vi "Facade.vi"(0 "Data In":T29={"Waveform"={"Type"=enum."Tone", "Tone"={"Frequency (kHz)"=0.0, "Last Freq"=0.0, "Last Phase"=0.0}, "Pulse Train"={"Pulse width (us)"=0.0, "Pulse rate (Hz)"=0.0, "Gap (ms)"=0.0, "Polarity"=enum."POS", "PT State"={"Template"=[], "Nperiod"=0, "Index"=0, "Pulse Rate (Hz)"=0.0, "Phase (cycles)"=0.0, "Noff"=0}, "Asynch"=FALSE}, "Noise"={"InvFilt"=FALSE, "Noise"=[], "CurPt"=0, "Aweight"=FALSE, "Seed"=0, "afile"=path ""}, "File"={"Filename"=path "", "Signal"=[], "Channel"=0, "stream"=FALSE, "offset"=0, "nreps"=0, "loops"=0, "Randomize"=FALSE, "order"=[], "Seed"=0, "Tokens"=0}, "FMSweep"={"Rate (oct/s)"=0.0, "Fmin (Hz)"=0.0, "Fmax (Hz)"=0.0, "Ramp (ms)"=0.0, "Linear"=FALSE}, "Chirp Train"={"Params"={"Fmin (kHz)"=4.0, "Fmax (kHz)"=64.0, "Compensate"=FALSE, "Duration (ms)"=2.0}, "Data"={"WF"=[]}}, "Complex Tone"={"Params"={"F0 (Hz)"=0.0, "Band"={"Flow (Hz)"=0.0, "Fhigh (Hz)"=0.0}, "Phase"=enum."Cosine", "Min F0 (Hz)"=0.0, "Max F0 (Hz)"=0.0, "ContinRandPhase"=FALSE, "Max peak factor"=inf, "Max mod depth"=2.0, "MinHarmNum"=0, "MaxHarmNum"=0, "Level Mode"=enum."per component", "% jitter"=0.0}, "Data"={"Ncomp"=0, "MinHarm"=0, "Phase"=[], "Amplitude"=[], "Npts/frame"=0, "Last F0"=0.0, "Fmin"=0.0, "Fmax"=0.0, "Lslope"=0.0, "randphase"=FALSE, "overall rms"=FALSE, "fmult"=[], "jittered"=FALSE}}, "Moving Ripple"={"Params"={"Fmin"=0.0, "Fmax"=0.0, "Density"=0.0, "Velocity"=0.0, "Depth"=0.0, "Phase"=0.0, "Comp/oct"=0}, "Data"={"Freq"=[], "A"=[], "phase"=[], "Phase"=0.0}}}, "Filter"={"Type"=enum."Lowpass", "CF (kHz)"=0.0, "BW (kHz)"=0.0, "Cascade"=FALSE, "Quadrature"=FALSE, "Scale Factor"=0.0, "Stages"=[], "Class"=enum."Elliptic", "Order"=0, "BWUnits"=enum."Linear"}, "Burst"={"Active"=FALSE, "Delay (ms)"=0.0, "Duration (ms)"=50.0, "Ramp (ms)"=5.0, "Rate (Hz)"=0.0, "Trepeat (ms)"=0.0, "Repeat"=FALSE}, "Level"={"Level"=0.0, "Units"=enum."dB atten", "Max"=0.0, "Multiplier"=0.0, "Cal File"=path "", "Cal"={"Freq (Hz)"=[], "Mag (dB SPL)"=[], "Phase (deg)"=[]}}, "Name"="", "Advanced"={"Rep Mask"="", "AltPol"=FALSE, "Var"="", "Expr"="", "Persist"=FALSE}, "SAM"={"Active"=FALSE, "Frequency (Hz)"=0.0, "Depth"=0.0, "Init Phase (cycles)"=0.0, "phase (degrees)"=0.0, "Asynch"=FALSE}} {"Filter"."Stages"."IIR Filter"."Forward Coefficients" format="%.4f"; "Filter"."Stages"."IIR Filter"."Reverse Coefficients" format="%.4f"}, 2 "Display State In":T27={"Update"=FALSE, "Show advanced"=FALSE, "Fs (Hz)"=100000.0, "Show persist"=FALSE}, 3 "Container State":T28) -> (6 "Data Out":T29={"Waveform"={"Type"=enum."Tone", "Tone"={"Frequency (kHz)"=0.0, "Last Freq"=0.0, "Last Phase"=0.0}, "Pulse Train"={"Pulse width (us)"=0.0, "Pulse rate (Hz)"=0.0, "Gap (ms)"=0.0, "Polarity"=enum."POS", "PT State"={"Template"=[], "Nperiod"=0, "Index"=0, "Pulse Rate (Hz)"=0.0, "Phase (cycles)"=0.0, "Noff"=0}, "Asynch"=FALSE}, "Noise"={"InvFilt"=FALSE, "Noise"=[], "CurPt"=0, "Aweight"=FALSE, "Seed"=0, "afile"=path ""}, "File"={"Filename"=path "", "Signal"=[], "Channel"=0, "stream"=FALSE, "offset"=0, "nreps"=0, "loops"=0, "Randomize"=FALSE, "order"=[], "Seed"=0, "Tokens"=0}, "FMSweep"={"Rate (oct/s)"=0.0, "Fmin (Hz)"=0.0, "Fmax (Hz)"=0.0, "Ramp (ms)"=0.0, "Linear"=FALSE}, "Chirp Train"={"Params"={"Fmin (kHz)"=4.0, "Fmax (kHz)"=64.0, "Compensate"=FALSE, "Duration (ms)"=2.0}, "Data"={"WF"=[]}}, "Complex Tone"={"Params"={"F0 (Hz)"=0.0, "Band"={"Flow (Hz)"=0.0, "Fhigh (Hz)"=0.0}, "Phase"=enum."Cosine", "Min F0 (Hz)"=0.0, "Max F0 (Hz)"=0.0, "ContinRandPhase"=FALSE, "Max peak factor"=inf, "Max mod depth"=2.0, "MinHarmNum"=0, "MaxHarmNum"=0, "Level Mode"=enum."per component", "% jitter"=0.0}, "Data"={"Ncomp"=0, "MinHarm"=0, "Phase"=[], "Amplitude"=[], "Npts/frame"=0, "Last F0"=0.0, "Fmin"=0.0, "Fmax"=0.0, "Lslope"=0.0, "randphase"=FALSE, "overall rms"=FALSE, "fmult"=[], "jittered"=FALSE}}, "Moving Ripple"={"Params"={"Fmin"=0.0, "Fmax"=0.0, "Density"=0.0, "Velocity"=0.0, "Depth"=0.0, "Phase"=0.0, "Comp/oct"=0}, "Data"={"Freq"=[], "A"=[], "phase"=[], "Phase"=0.0}}}, "Filter"={"Type"=enum."Lowpass", "CF (kHz)"=0.0, "BW (kHz)"=0.0, "Cascade"=FALSE, "Quadrature"=FALSE, "Scale Factor"=0.0, "Stages"=[], "Class"=enum."Elliptic", "Order"=0, "BWUnits"=enum."Linear"}, "Burst"={"Active"=FALSE, "Delay (ms)"=0.0, "Duration (ms)"=50.0, "Ramp (ms)"=5.0, "Rate (Hz)"=0.0, "Trepeat (ms)"=0.0, "Repeat"=FALSE}, "Level"={"Level"=0.0, "Units"=enum."dB atten", "Max"=0.0, "Multiplier"=0.0, "Cal File"=path "", "Cal"={"Freq (Hz)"=[], "Mag (dB SPL)"=[], "Phase (deg)"=[]}}, "Name"="", "Advanced"={"Rep Mask"="", "AltPol"=FALSE, "Var"="", "Expr"="", "Persist"=FALSE}, "SAM"={"Active"=FALSE, "Frequency (Hz)"=0.0, "Depth"=0.0, "Init Phase (cycles)"=0.0, "phase (degrees)"=0.0, "Asynch"=FALSE}} {"Filter"."Stages"."IIR Filter"."Forward Coefficients" format="%.4f"; "Filter"."Stages"."IIR Filter"."Reverse Coefficients" format="%.4f"}, 7 "Display State Out":T27={"Update"=FALSE, "Show advanced"=FALSE, "Fs (Hz)"=100000.0, "Show persist"=FALSE}, 8 "Action":T26)   [LabVIEW 2020, in "Stimulus Channel (Full).xctl"]
uses:
  Stimulus Channel (Full).xctl
  Full Stimulus Channel Data.ctl
  Waveform XCtl/Waveform Data.ctl
  Waveform XCtl/Waveform Enum.ctl
  Waveform VIs/Tone VIs/Tone Params.ctl
  Waveform VIs/Pulse Train VIs/Pulse Train Params.ctl
  Waveform VIs/Pulse Train VIs/Pulse Polarity.ctl
  Waveform VIs/Pulse Train VIs/PT-Continuous State.ctl
  Waveform VIs/Noise VIs/Noise Params.ctl
  Waveform VIs/File VIs/StimFile-Params.ctl
  Waveform VIs/FM Sweep VIs/FM Sweep Params.ctl
  Waveform VIs/Chirp Train VIs/Chirp Train.ctl
  Waveform VIs/Chirp Train VIs/Chirp Train Params.ctl
  Waveform VIs/Complex Tone VIs/CT-Params.ctl
  Waveform VIs/Complex Tone VIs/CT-Phase Enum.ctl
  Waveform VIs/Complex Tone VIs/CT-Runtime Data.ctl
  Waveform VIs/Moving Ripple VIs/Moving Ripple.ctl
  Waveform VIs/Moving Ripple VIs/Moving Ripple.Params.ctl
  Waveform VIs/Moving Ripple VIs/Moving Ripple.Data.ctl
  Advanced Filter XCtl/Filter Data.ctl
  Filter VIs/Filter-Bandwidth Units.ctl
  Burst XCtl/Burst Data.ctl
  Level XCtl/Level Data.ctl
  Level XCtl/Level Units.ctl
  Advanced Options XCtl/Advanced Stimulus Options.ctl
  Modulation VIs/SAM VIs/SAM Params.ctl
  <vilib>/_xctls/Container State.ctl
  State.ctl
  <vilib>/_xctls/Action.ctl
  Advanced Filter XCtl/Advanced Filter XCtl.xctl
  Level XCtl/Level XCtl.xctl
  Burst XCtl/Burst Control.xctl
  Waveform XCtl/Waveform XCtl.xctl
  Advanced Options XCtl/Advanced Stimulus Options.xctl
  <vilib>/_xctls/XControlSupport.lvlib
panel:
  out "SAM-dependent display":bool
  out "waveform-dependent display":bool
  out "update max level":bool
  in  "Tab Control":T1(tab)=enum."Filtering"
  in  "Waveform":T18(xcontrol)
  in  "Level":T20(xcontrol)
  in  "Gate":T21(xcontrol)
  in  "SAM":T22
  in  "Filter":T24(xcontrol)
  in  "Advanced":T25(xcontrol)
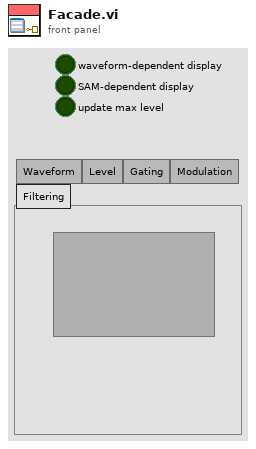
[diagram p1: front panel]
types:
  T1 = enum32{"Waveform", "Level", "Gating", "Modulation", "Filtering", "Advanced"}
  T2 = typedef "Waveform Enum.ctl" = enum16{"OFF", "Tone", "Noise", "Pulse Train", "File", "FM Sweep", "Chirp Train", "Complex Tone", "FM Tone", "Moving Ripple"}
  T3 = typedef "Tone Params.ctl" = cluster{"Frequency (kHz)":dbl, "Last Freq":dbl, "Last Phase":dbl}
  T4 = typedef "Pulse Train Params.ctl" = cluster{"Pulse width (us)":dbl, "Pulse rate (Hz)":dbl, "Gap (ms)":dbl, "Polarity":T5, "PT State":T6, "Asynch":bool}
  T5 = typedef "Pulse Polarity.ctl" = enum16{"POS", "NEG", "POS-NEG", "NEG-POS"}
  T6 = typedef "PT-Continuous State.ctl" = cluster{"Template":dbl[], "Nperiod":i32, "Index":i32, "Pulse Rate (Hz)":dbl, "Phase (cycles)":dbl, "Noff":i32}
  T7 = typedef "Noise Params.ctl" = cluster{"InvFilt":bool, "Noise":dbl[], "CurPt":i32, "Aweight":bool, "Seed":i32, "afile":path}
  T8 = typedef "StimFile-Params.ctl" = cluster{"Filename":path, "Signal":dbl[], "Channel":i32, "stream":bool, "offset":i32, "nreps":i32, "loops":i32, "Randomize":bool, "order":i32[], "Seed":i32, "Tokens":i32}
  T9 = typedef "FM Sweep Params.ctl" = cluster{"Rate (oct/s)":dbl, "Fmin (Hz)":dbl, "Fmax (Hz)":dbl, "Ramp (ms)":dbl, "Linear":bool}
  T10 = typedef "Chirp Train.ctl" = cluster{"Params":T11, "Data":cluster{"WF":dbl[]}}
  T11 = typedef "Chirp Train Params.ctl" = cluster{"Fmin (kHz)":dbl, "Fmax (kHz)":dbl, "Compensate":bool, "Duration (ms)":dbl}
  T12 = typedef "CT-Params.ctl" = cluster{"F0 (Hz)":dbl, "Band":cluster{"Flow (Hz)":dbl, "Fhigh (Hz)":dbl}, "Phase":T13, "Min F0 (Hz)":dbl, "Max F0 (Hz)":dbl, "ContinRandPhase":bool, "Max peak factor":dbl, "Max mod depth":dbl, "MinHarmNum":i32, "MaxHarmNum":i32, "Level Mode":enum16{"per component", "overall rms"}, "% jitter":dbl}
  T13 = typedef "CT-Phase Enum.ctl" = enum16{"Cosine", "Random", "Alternating"}
  T14 = typedef "CT-Runtime Data.ctl" = cluster{"Ncomp":i32, "MinHarm":i32, "Phase":dbl[], "Amplitude":dbl[], "Npts/frame":i32, "Last F0":dbl, "Fmin":dbl, "Fmax":dbl, "Lslope":dbl, "randphase":bool, "overall rms":bool, "fmult":dbl[], "jittered":bool}
  T15 = typedef "Moving Ripple.ctl" = cluster{"Params":T16, "Data":T17}
  T16 = typedef "Moving Ripple.Params.ctl" = cluster{"Fmin":dbl, "Fmax":dbl, "Density":dbl, "Velocity":dbl, "Depth":dbl, "Phase":dbl, "Comp/oct":i32}
  T17 = typedef "Moving Ripple.Data.ctl" = cluster{"Freq":dbl[], "A":dbl[], "phase":dbl[], "Phase":dbl}
  T18 = cluster{"Type":T2, "Tone":T3, "Pulse Train":T4, "Noise":T7, "File":T8, "FMSweep":T9, "Chirp Train":T10, "Complex Tone":cluster{"Params":T12, "Data":T14}, "Moving Ripple":T15}
  T19 = typedef "Level Units.ctl" = enum16{"dB atten", "dB SPL", "dB re 1 Vrms", "dB V/Hz½", "mW", "dB HL", "Volts", "dB mW"}
  T20 = cluster{"Level":dbl, "Units":T19, "Max":dbl, "Multiplier":dbl, "Cal File":path, "Cal":cluster{"Freq (Hz)":dbl[], "Mag (dB SPL)":dbl[], "Phase (deg)":dbl[]}}
  T21 = cluster{"Active":bool, "Delay (ms)":dbl, "Duration (ms)":dbl, "Ramp (ms)":dbl, "Rate (Hz)":dbl, "Trepeat (ms)":dbl, "Repeat":bool}
  T22 = cluster{"Active":bool, "Frequency (Hz)":dbl, "Depth (0-1)":dbl, "Phase (cycles)":dbl, "phase":dbl, "Asynch":bool}
  T23 = typedef "Filter-Bandwidth Units.ctl" = enum16{"Linear", "Octaves", "Min-Max"}
  T24 = cluster{"Type":enum16{"Lowpass", "Highpass", "Bandpass", "Bandstop", "OFF"}, "CF (kHz)":dbl, "BW (kHz)":dbl, "Cascade":bool, "Quadrature":bool, "Scale Factor":dbl, "Stages":cluster{"IIR Filter":cluster{"filter structure":enum32{"IIR 2nd Order", "IIR 4th Order"}, "Reverse Coefficients":dbl[], "Forward Coefficients":dbl[]}, "State":dbl[]}[], "Class":enum16{"Elliptic", "Butterworth"}, "Order":i32, "BWUnits":T23}
  T25 = cluster{"Rep Mask":string, "AltPol":bool, "Var":string, "Expr":string, "Persist":bool}
  T26 = typedef "XControlSupport.lvlib/Action.ctl" = cluster{"Data Changed?":bool, "State Changed?":bool, "Action Name":string}
  T27 = typedef "Stimulus Channel (Full).xctl/State.ctl" = cluster{"Update":bool, "Show advanced":bool, "Fs (Hz)":dbl, "Show persist":bool}
  T28 = typedef "XControlSupport.lvlib/Container State.ctl" = cluster{"Indicator?":bool, "Run Mode?":bool, " Refnum":refnum<vi>}
  T29 = typedef "Stimulus Channel (Full).xctl/Full Stimulus Channel Data.ctl" = cluster{"Waveform":T30, "Filter":T31, "Burst":T32, "Level":T33, "Name":string, "Advanced":T34, "SAM":T35}
  T30 = typedef "Waveform XCtl.xctl/Waveform Data.ctl" = cluster{"Type":T2, "Tone":T3, "Pulse Train":T4, "Noise":T7, "File":T8, "FMSweep":T9, "Chirp Train":T10, "Complex Tone":cluster{"Params":T12, "Data":T14}, "Moving Ripple":T15}
  T31 = typedef "Advanced Filter XCtl.xctl/Filter Data.ctl" = cluster{"Type":enum16{"Lowpass", "Highpass", "Bandpass", "Bandstop", "OFF"}, "CF (kHz)":dbl, "BW (kHz)":dbl, "Cascade":bool, "Quadrature":bool, "Scale Factor":dbl, "Stages":cluster{"IIR Filter":cluster{"filter structure":enum32{"IIR 2nd Order", "IIR 4th Order"}, "Reverse Coefficients":dbl[], "Forward Coefficients":dbl[]}, "State":dbl[]}[], "Class":enum16{"Elliptic", "Butterworth"}, "Order":i32, "BWUnits":T23}
  T32 = typedef "Burst Control.xctl/Burst Data.ctl" = cluster{"Active":bool, "Delay (ms)":dbl, "Duration (ms)":dbl, "Ramp (ms)":dbl, "Rate (Hz)":dbl, "Trepeat (ms)":dbl, "Repeat":bool}
  T33 = typedef "Level XCtl.xctl/Level Data.ctl" = cluster{"Level":dbl, "Units":T19, "Max":dbl, "Multiplier":dbl, "Cal File":path, "Cal":cluster{"Freq (Hz)":dbl[], "Mag (dB SPL)":dbl[], "Phase (deg)":dbl[]}}
  T34 = typedef "Advanced Stimulus Options.xctl/Advanced Stimulus Options.ctl" = cluster{"Rep Mask":string, "AltPol":bool, "Var":string, "Expr":string, "Persist":bool}
  T35 = typedef "SAM Params.ctl" = cluster{"Active":bool, "Frequency (Hz)":dbl, "Depth":dbl, "Init Phase (cycles)":dbl, "phase (degrees)":dbl, "Asynch":bool}
  T36 = enum32{"Waveform", "Level", "Gating", "Modulation", "Filtering"}
  T37 = enum16{"Lowpass", "Highpass", "Bandpass", "Bandstop", "OFF"}
  T38 = enum8{"Enabled", "Disabled", "Disabled and Grayed Out"}
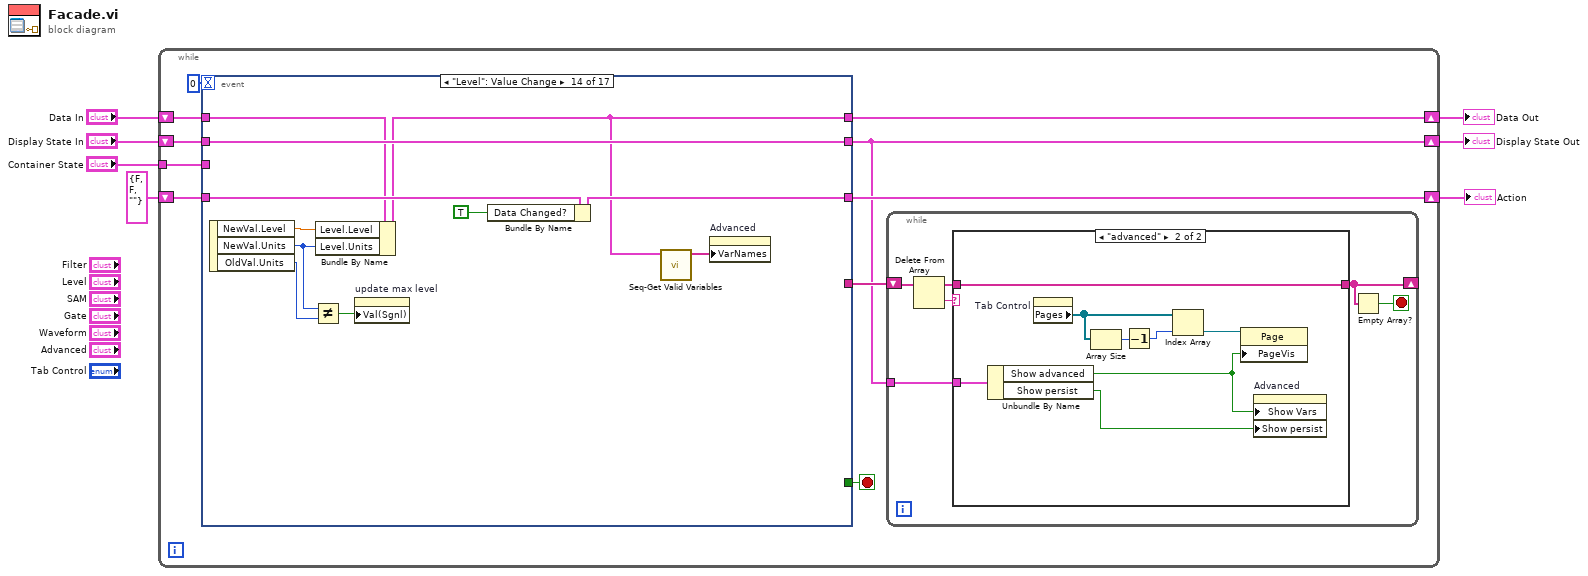
[diagram p0: block diagram]
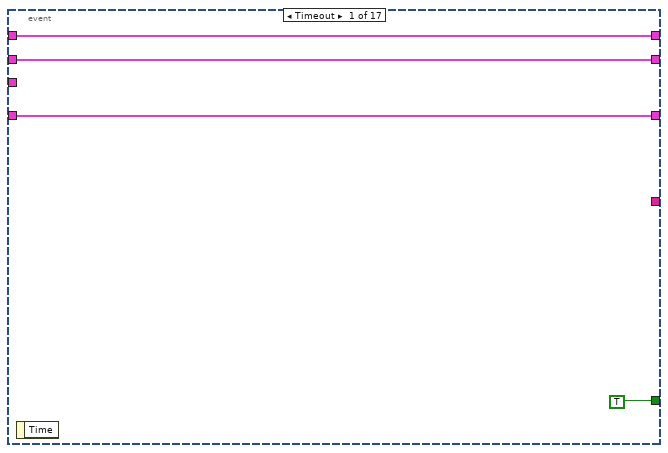
[diagram p3: hidden frame]
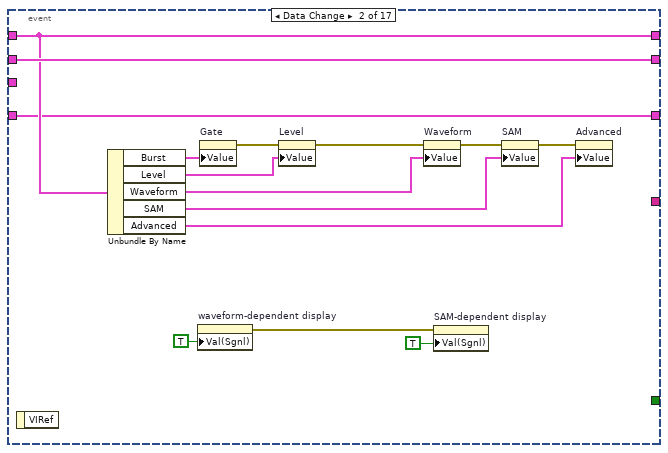
[diagram p4: hidden frame]
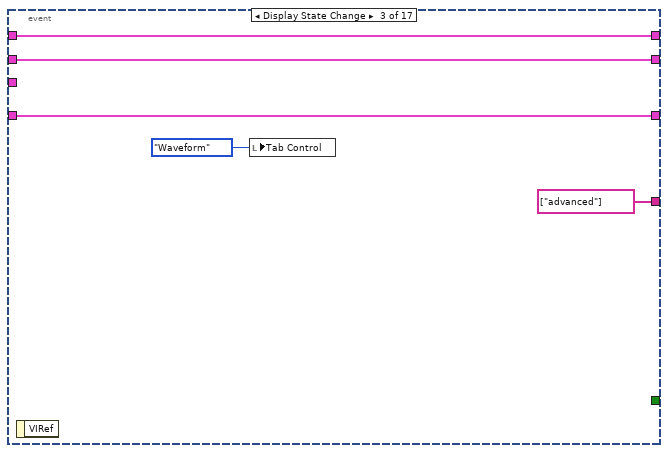
[diagram p5: hidden frame]
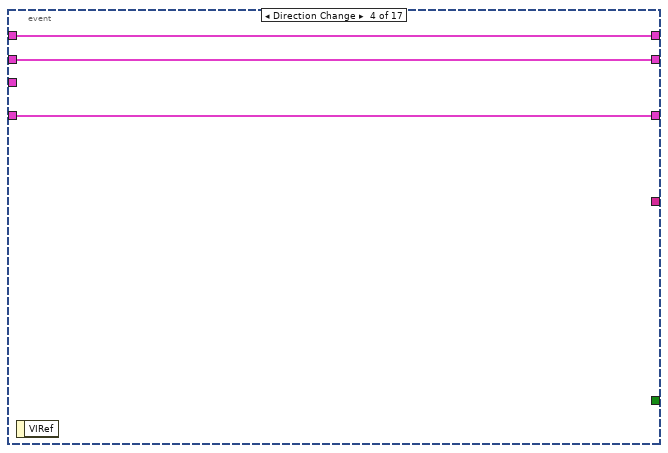
[diagram p6: hidden frame]
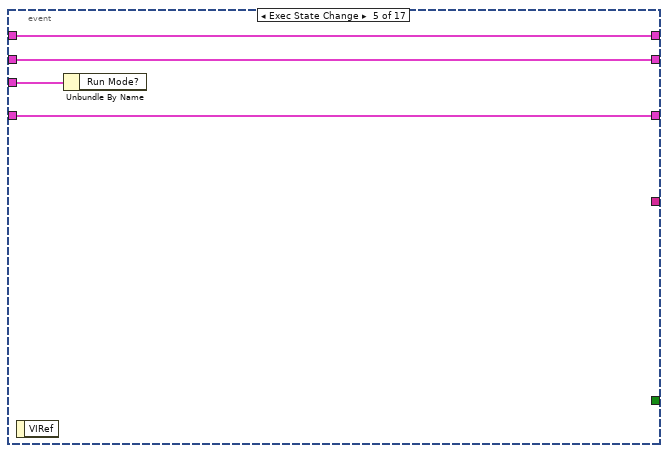
[diagram p7: hidden frame]
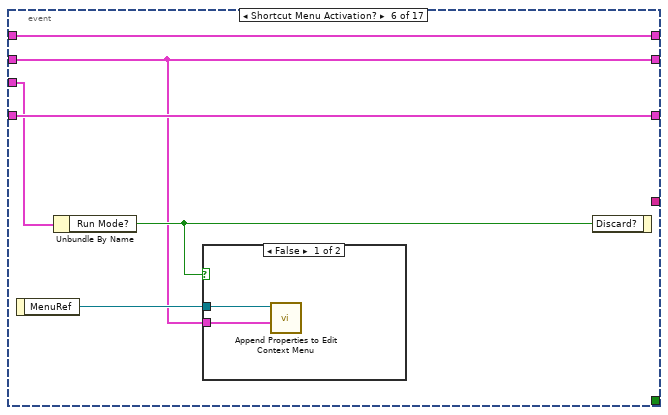
[diagram p8: hidden frame]
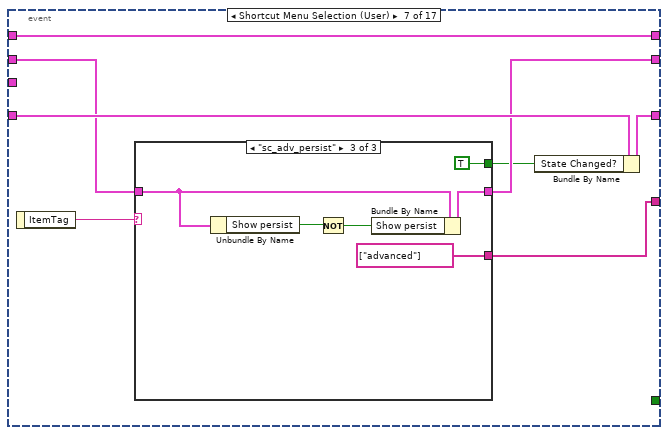
[diagram p10: hidden frame]
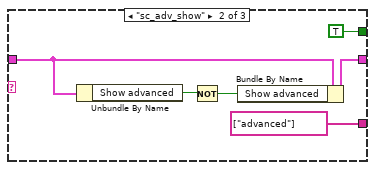
[diagram p12: hidden frame]
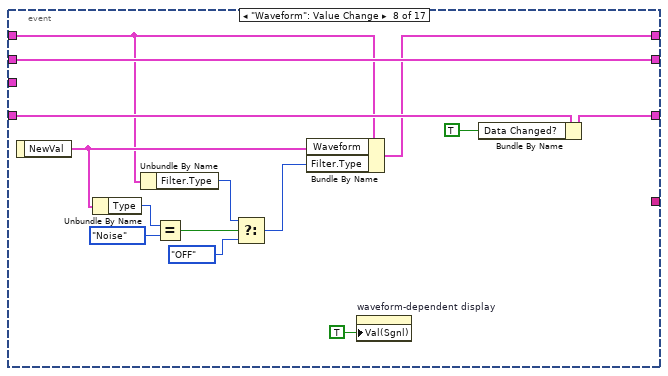
[diagram p13: hidden frame]
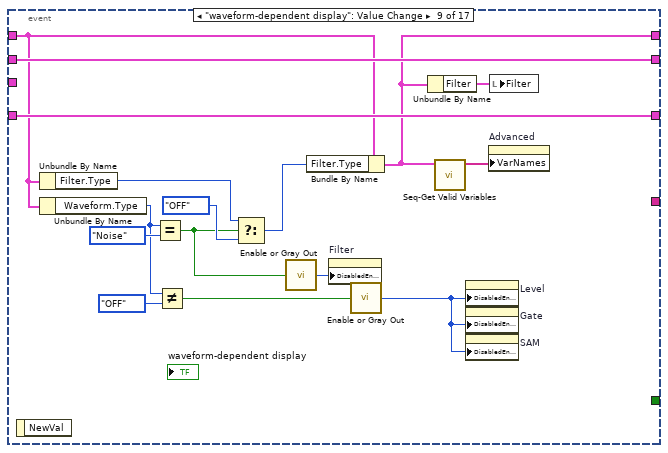
[diagram p14: hidden frame]
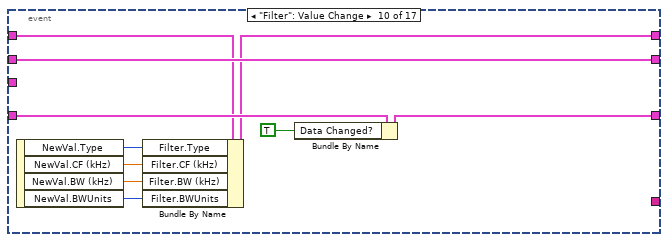
[diagram p15: hidden frame]
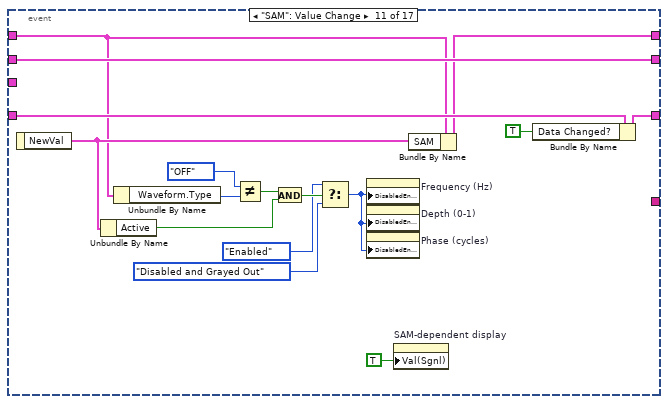
[diagram p16: hidden frame]
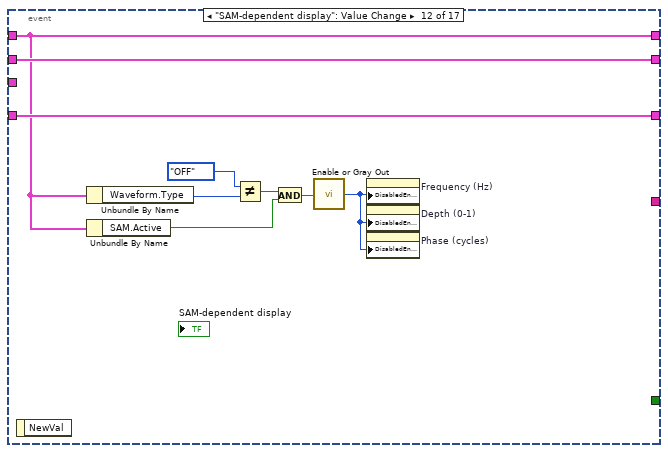
[diagram p17: hidden frame]
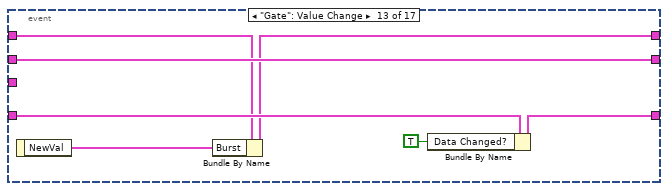
[diagram p18: hidden frame]
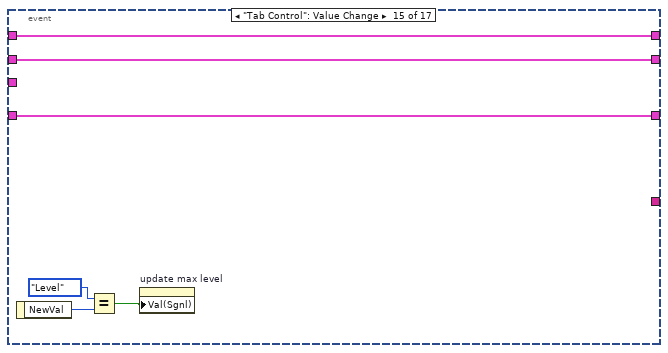
[diagram p19: hidden frame]
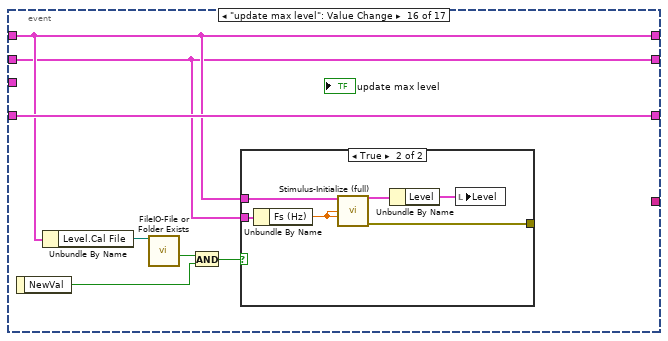
[diagram p20: hidden frame]
diagram:
  n1 = while {
    shift-right: [w8] -> w4
    shift-left: "Display State In" -> [w17]
    tunnel: "Container State" -> [w14]
    shift-right: [w12] -> w7
    shift-left: "Data In" -> [w13]
    shift-right: [w10] -> w2
    shift-left: T26 {"Data Changed?"=FALSE, "State Changed?"=FALSE, "Action Name"=""} ("Action") -> [w11]
    stop <- w16 stop-if-true
    n2 = event shown="[13] \"Level\": Value Change" {
      selector: _ -> [_ _ _ _ _ _ _ _ _ _ _ _ _ _ _ _ _]
      dyn-events: _ -> [_ _ _ _ _ _ _ _ _ _ _ _ _ _ _ _ _]
      timeout: 0 -> [_ _ _ _ _ _ _ _ _ _ _ _ _ _ _ _ _]
      tunnel: w17 -> [w34 w51 w53 w59 w62 w64 w76 w103 w121 w129 w148 w157 w162 w172 w177 w183 w198]
      tunnel: [w34 w51 w53 w59 w62 w64 w75 w103 w121 w129 w148 w157 w162 w172 w177 w183 w198] -> w8
      tunnel: [TRUE _ _ _ _ _ _ _ _ _ _ _ _ _ _ _ _] -> w16
      tunnel: w14 -> [_ _ _ _ w63 w67 _ _ _ _ _ _ _ _ _ _ _]
      tunnel: w13 -> [w33 w50 w56 w58 w61 w69 w79 w95 w109 w128 w142 w151 w161 w171 w178 w184 w197]
      tunnel: [w33 w50 w56 w58 w61 w69 w79 w94 w108 w127 w146 w151 w160 w165 w178 w184 w196] -> w12
      tunnel: [w35 w49 w55 w57 w60 w68 w74 w104 w122 w130 w145 w156 w163 w173 w181 w188 w199] -> w10
      tunnel: w11 -> [w35 w49 w55 w57 w60 w68 w78 w106 w122 w132 w147 w156 w164 w175 w181 w188 w201]
      tunnel: [_ _ string[] ["advanced"] _ _ _ w72 _ _ _ _ _ _ _ _ _ _] -> w9
      event Timeout {
        n3 = event-data() -> ()  [unwired: 1 in, 1 out]
      }
      event Data Change {
        n4 = event-data() -> ()  [unwired: 1 in, 1 out]
        n5 = Unbundle By Name(w50) -> ("Burst"=w43:T32, "Level"=w47:T33, "Waveform"=w46:T30, "SAM"=w45:T35, "Advanced"=w44:T34)
        n6 = property on="waveform-dependent display" class="Bool (strict)"("Val(Sgnl)"=TRUE ("Value (Signaling)")) -> (error out=w40:errorcluster)  [unwired: 2 in, 1 out]
        n7 = property on="Gate" class="Burst Control (strict)"("Value"=w43) -> (error out=w48:errorcluster)  [unwired: 2 in, 1 out]
        n8 = property on="Level" class="Level XCtl (strict)"(error in=w48, "Value"=w47) -> (error out=w42:errorcluster)  [unwired: 1 in, 1 out]
        n9 = property on="Waveform" class="Waveform XCtl (strict)"(error in=w42, "Value"=w46) -> (error out=w41:errorcluster)  [unwired: 1 in, 1 out]
        n10 = property on="SAM-dependent display" class="Bool (strict)"(error in=w40, "Val(Sgnl)"=TRUE ("Value (Signaling)")) -> ()  [unwired: 1 in, 2 out]
        n11 = property on="SAM" class="Clust (strict)"(error in=w41, "Value"=w45) -> (error out=w39:errorcluster)  [unwired: 1 in, 1 out]
        n12 = property on="Advanced" class="Advanced Stimulus Options (stri"(error in=w39, "Value"=w44) -> ()  [unwired: 1 in, 2 out]
      }
      event Display State Change {
        n13 = event-data() -> ()  [unwired: 1 in, 1 out]
        n14 = local write "Tab Control"(T36."Waveform" ("Tab Control")) -> ()
      }
      event Direction Change {
        n15 = event-data() -> ()  [unwired: 1 in, 1 out]
      }
      event Exec State Change {
        n16 = event-data() -> ()  [unwired: 1 in, 1 out]
        n17 = Unbundle By Name(w63) -> ()  [unwired: 1 out]
      }
      event Shortcut Menu Activation? {
        n18 = event-data() -> ("MenuRef"=w65:refnum<k9>)  [unwired: 1 in]
        n19 = Unbundle By Name(w67) -> ("Run Mode?"=w66:bool)
        n20 = case shown="False" w66 {
          tunnel: w65 -> [w71 _]
          tunnel: w64 -> [w70 _]
          frame False {
            n21 = call "Append Properties to Edit Context Menu.vi"("State"=w70, "Menu in"=w71) -> ()  [unwired: 10 in]
          }
          frame True {
          }
        }
        n22 = event-data("Discard?"=w66) -> ()  [unwired: 1 in, 1 out]
      }
      event Shortcut Menu Selection (User) {
        n23 = event-data() -> ("ItemTag"=w77:string)  [unwired: 1 in]
        n24 = case shown="\"sc_adv_persist\"" w77 {
          tunnel: w76 -> [w80 w86 w92]
          tunnel: [w80 w85 w91] -> w75
          tunnel: [_ TRUE TRUE] -> w73
          tunnel: [_ string[] ["advanced"] string[] ["advanced"]] -> w72
          frame "", Default {
          }
          frame "sc_adv_show" {
            n25 = Unbundle By Name(w86) -> ("Show advanced"=w84:bool)
            n26 = Not(x=w84) -> (.not. x?=w83:bool)
            n27 = Bundle By Name(cluster=w86, "Show advanced"=w83) -> (w85:T27)
          }
          frame "sc_adv_persist" {
            n28 = Unbundle By Name(w92) -> ("Show persist"=w90:bool)
            n29 = Not(x=w90) -> (.not. x?=w89:bool)
            n30 = Bundle By Name(cluster=w92, "Show persist"=w89) -> (w91:T27)
          }
        }
        n31 = Bundle By Name(cluster=w78, "State Changed?"=w73) -> (w74:T26)
      }
      event "Waveform": Value Change {
        n32 = event-data() -> ("NewVal"=w102:T18)  [unwired: 1 in]
        n33 = Unbundle By Name(w102) -> ("Type"=w96:T2)
        n34 = Unbundle By Name(w95) -> ("Filter.Type"=w100:T37)
        n35 = Equal?(x=w96, y=Waveform_Enum."Noise") -> (x = y?=w97:bool)
        n36 = Select(t=w100, s=w97, f=T37."OFF") -> (s? t:f=w98:T37)
        n37 = Bundle By Name(cluster=w95, "Waveform"=w102, "Filter.Type"=w98) -> (w94:T29)
        n38 = property on="waveform-dependent display" class="Bool (strict)"("Val(Sgnl)"=TRUE ("Value (Signaling)")) -> ()  [unwired: 2 in, 2 out]
        n39 = Bundle By Name(cluster=w106, "Data Changed?"=TRUE) -> (w104:T26)
      }
      event "waveform-dependent display": Value Change {
        n40 = event-data() -> ()  [unwired: 1 in, 1 out]
        n41 = Unbundle By Name(w109) -> ("Filter.Type"=w119:T37)
        n42 = Unbundle By Name(w109) -> ("Waveform.Type"=w115:T2)
        n43 = Equal?(x=w115, y=Waveform_Enum."Noise") -> (x = y?=w111:bool)
        n44 = Not Equal?(x=w115, y=Waveform_Enum."OFF") -> (x != y?=w113:bool)
        n45 = Select(t=w119, s=w111, f=T37."OFF") -> (s? t:f=w117:T37)
        n46 = call "Enable or Gray Out.vi"("Boolean"=w111) -> ("Disabled"=w110:T38)
        n47 = Bundle By Name(cluster=w109, "Filter.Type"=w117) -> (w108:T29)
        n48 = property on="Filter" class="Advanced Filter XCtl (strict)"("DisabledEnum"=w110) -> ()  [unwired: 2 in, 2 out]
        n49 = call "Enable or Gray Out.vi"("Boolean"=w113) -> ("Disabled"=w112:T38)
        n50 = Unbundle By Name(w108) -> ("Filter"=w116:T31)
        n51 = call "Seq-Get Valid Variables.vi"("StimChan"=w108) -> ("VarNames"=w107:string[])  [unwired: 10 in]
        n52 = property on="Level" class="Level XCtl (strict)"("DisabledEnum"=w112) -> ()  [unwired: 2 in, 2 out]
        n53 = property on="Gate" class="Burst Control (strict)"("DisabledEnum"=w112) -> ()  [unwired: 2 in, 2 out]
        n54 = property on="SAM" class="Clust (strict)"("DisabledEnum"=w112) -> ()  [unwired: 2 in, 2 out]
        n55 = property on="Advanced" class="Advanced Stimulus Options (stri"("VarNames"=w107) -> ()  [unwired: 2 in, 2 out]
        n56 = local write "Filter"(w116) -> ()
      }
      event "Filter": Value Change {
        n57 = event-data() -> ("NewVal.Type"=w126:T37, "NewVal.CF (kHz)"=w125:dbl, "NewVal.BW (kHz)"=w124:dbl, "NewVal.BWUnits"=w123:T23)  [unwired: 1 in]
        n58 = Bundle By Name(cluster=w128, "Filter.Type"=w126, "Filter.CF (kHz)"=w125, "Filter.BW (kHz)"=w124, "Filter.BWUnits"=w123) -> (w127:T29)
        n59 = Bundle By Name(cluster=w132, "Data Changed?"=TRUE) -> (w130:T26)
      }
      event "SAM": Value Change {
        n60 = event-data() -> ("NewVal"=w143:T22)  [unwired: 1 in]
        n61 = Unbundle By Name(w143) -> ("Active"=w138:bool)
        n62 = Unbundle By Name(w142) -> ("Waveform.Type"=w141:T2)
        n63 = Not Equal?(x=Waveform_Enum."OFF", y=w141) -> (x != y?=w139:bool)
        n64 = And(x=w139, y=w138) -> (x .and. y?=w137:bool)
        n65 = Select(t=T38."Enabled" ("Disabled"), s=w137, f=T38."Disabled and Grayed Out" ("Disabled")) -> (s? t:f=w134:T38)
        n66 = property on="Frequency (Hz)" class="DigNum (strict)"("DisabledEnum"=w134) -> ()  [unwired: 2 in, 2 out]
        n67 = property on="Depth (0-1)" class="DigNum (strict)"("DisabledEnum"=w134) -> ()  [unwired: 2 in, 2 out]
        n68 = property on="Phase (cycles)" class="DigNum (strict)"("DisabledEnum"=w134) -> ()  [unwired: 2 in, 2 out]
        n69 = property on="SAM-dependent display" class="Bool (strict)"("Val(Sgnl)"=TRUE ("Value (Signaling)")) -> ()  [unwired: 2 in, 2 out]
        n70 = Bundle By Name(cluster=w142, "SAM"=w143) -> (w146:T29)
        n71 = Bundle By Name(cluster=w147, "Data Changed?"=TRUE) -> (w145:T26)
      }
      event "SAM-dependent display": Value Change {
        n72 = event-data() -> ()  [unwired: 1 in, 1 out]
        n73 = Unbundle By Name(w151) -> ("Waveform.Type"=w155:T2)
        n74 = Unbundle By Name(w151) -> ("SAM.Active"=w152:bool)
        n75 = Not Equal?(x=Waveform_Enum."OFF", y=w155) -> (x != y?=w153:bool)
        n76 = And(x=w153, y=w152) -> (x .and. y?=w150:bool)
        n77 = call "Enable or Gray Out.vi"("Boolean"=w150) -> ("Disabled"=w149:T38)
        n78 = property on="Frequency (Hz)" class="DigNum (strict)"("DisabledEnum"=w149) -> ()  [unwired: 2 in, 2 out]
        n79 = property on="Depth (0-1)" class="DigNum (strict)"("DisabledEnum"=w149) -> ()  [unwired: 2 in, 2 out]
        n80 = property on="Phase (cycles)" class="DigNum (strict)"("DisabledEnum"=w149) -> ()  [unwired: 2 in, 2 out]
      }
      event "Gate": Value Change {
        n81 = event-data() -> ("NewVal"=w159:T21)  [unwired: 1 in]
        n82 = Bundle By Name(cluster=w161, "Burst"=w159) -> (w160:T29)
        n83 = Bundle By Name(cluster=w164, "Data Changed?"=TRUE) -> (w163:T26)
      }
      event "Level": Value Change {
        n84 = event-data() -> ("NewVal.Level"=w170:dbl, "NewVal.Units"=w169:T19, "OldVal.Units"=w168:T19)  [unwired: 1 in]
        n85 = Not Equal?(x=w169, y=w168) -> (x != y?=w167:bool)
        n86 = Bundle By Name(cluster=w171, "Level.Level"=w170, "Level.Units"=w169) -> (w165:T29)
        n87 = property on="update max level" class="Bool (strict)"("Val(Sgnl)"=w167) -> ()  [unwired: 2 in, 2 out]
        n88 = Bundle By Name(cluster=w175, "Data Changed?"=TRUE) -> (w173:T26)
        n89 = call "Seq-Get Valid Variables.vi"("StimChan"=w165) -> ("VarNames"=w166:string[])  [unwired: 10 in]
        n90 = property on="Advanced" class="Advanced Stimulus Options (stri"("VarNames"=w166) -> ()  [unwired: 2 in, 2 out]
      }
      event "Tab Control": Value Change {
        n91 = event-data() -> ("NewVal"=w180:T1)  [unwired: 1 in]
        n92 = Equal?(x=T1."Level", y=w180) -> (x = y?=w176:bool)
        n93 = property on="update max level" class="Bool (strict)"("Val(Sgnl)"=w176) -> ()  [unwired: 2 in, 2 out]
      }
      event "update max level": Value Change {
        n94 = event-data() -> ("NewVal"=w182:bool)  [unwired: 1 in]
        n95 = Unbundle By Name(w184) -> ("Level.Cal File"=w187:path)
        n96 = call "FileIO-File or Folder Exists.vi"("path"=w187) -> ("Exists?"=w186:bool)  [unwired: 7 in, 3 out]
        n97 = And(x=w186, y=w182) -> (x .and. y?=w185:bool)
        n98 = case shown="True" w185 {
          tunnel: w184 -> [_ w194]
          tunnel: [_ w191] -> _
          tunnel: w183 -> [_ w190]
          frame False {
          }
          frame True {
            n99 = Unbundle By Name(w190) -> ("Fs (Hz)"=w189:dbl)
            n100 = call "Stimulus-Initialize (full).vi"("Stimulus Channel"=w194, "Sampling rate (Hz)"=w189, "Npts"=w189) -> ("Stimulus Channel out"=w193:T29, "error out"=w191:errorcluster)  [unwired: 10 in, 1 out]
            n101 = Unbundle By Name(w193) -> ("Level"=w192:T33)
            n102 = local write "Level"(w192) -> ()
          }
        }
      }
      event "Advanced": Value Change {
        n103 = event-data() -> ("NewVal"=w195:T25)  [unwired: 1 in]
        n104 = Bundle By Name(cluster=w197, "Advanced"=w195) -> (w196:T29)
        n105 = Bundle By Name(cluster=w201, "Data Changed?"=TRUE) -> (w199:T26)
      }
    }
    n106 = while {
      shift-right: [w20] -> _
      shift-left: w9 -> [w23]
      tunnel: w8 -> [w18]
      stop <- w19 stop-if-true
      n107 = Delete From Array(array=w23) -> (deleted portion=w21:string, array with subset deleted=w22:string[])  [unwired: 2 in]
      n108 = case shown="\"advanced\"" w21 {
        tunnel: w22 -> [w24 w32]
        tunnel: [w24 w32] -> w20
        tunnel: w18 -> [_ w26]
        frame "", Default {
        }
        frame "advanced" {
          n109 = Unbundle By Name(w26) -> ("Show advanced"=w31:bool, "Show persist"=w25:bool)
          n110 = property on="Tab Control" class="TabCtl (strict)"() -> ("Pages"=w27:refnum<vi>[])  [unwired: 2 in, 2 out]
          n111 = Array Size(array=w27) -> (size(s)=w28:i32)
          n112 = Decrement(x=w28) -> (x-1=w29:i32)
          n113 = Index Array(array=w27, index=w29) -> (element=w30:refnum<vi>)
          n114 = property class="Page"(reference=w30, "PageVis"=w31) -> ()  [unwired: 1 in, 2 out]
          n115 = property on="Advanced" class="Advanced Stimulus Options (stri"("Show Vars"=w31, "Show persist"=w25) -> ()  [unwired: 2 in, 2 out]
        }
      }
      n116 = Empty Array?(array=w20) -> (empty?=w19:bool)
    }
  }
  "Display State Out" <- w4
  "Data Out" <- w7
  "Action" <- w2
